vi "Close.vi"(0 "eye scan point iterator":refnum<class "niHighSpeedSerial N Point Eye Scan Point Iterator v1 Host.lvclass">, 11 "error in":errorcluster) -> (15 "error out":errorcluster)   [LabVIEW 2014, in "niHighSpeedSerial N Point Eye Scan Point Iterator v1 Host.lvclass"]
doc: "Closes the Eye Scan Point Iterator and frees resources.\n\n<B>Input Parameters</B>\n\n<B>eye scan point iterator</B> is the incoming wire for the Eye Scan Point Iterator class object\n\n<B>error in</B> describes error conditions that occur before this node runs. This input provides standard 'error in' functionality.\n\n<B>Output Parameters</B>\n\n<B>error out</B> contains error information. This output provides standard 'error out' functionality."
uses:
  <instrlib>/niHighSpeedSerial/Eye Scan/v1/Host/Impl/N Pt Iter/niHighSpeedSerial N Point Eye Scan Point Iterator v1 Host.lvclass
  <instrlib>/niHighSpeedSerial/Eye Scan/v1/Host/Impl/Eye Scan Point Iterator/niHighSpeedSerial Eye Scan Point Iterator v1 Host.lvclass
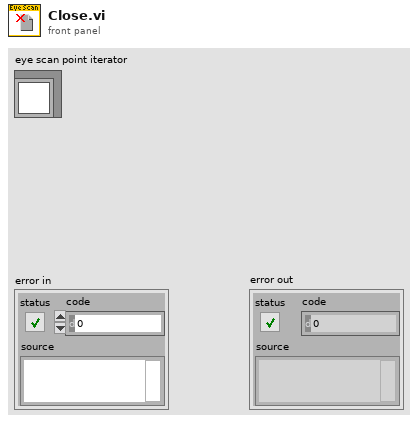
[diagram p1: front panel]
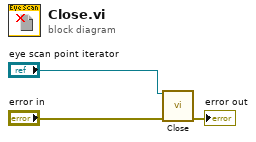
[diagram p0: block diagram]
diagram:
  n1 = call-parent "Close.vi"("eye scan point iterator"="eye scan point iterator", "error in"="error in") -> ("error out"=→"error out":errorcluster)  [unwired: 13 in]
